vi "SetParam.vi"(8 "error in (no error)":errorcluster caption="entrée d'erreur (pas d'erreur)", 10 "manhattan_distances":cluster{"sum_over_features":bool}={"sum_over_features"=TRUE}, 11 "Manhattan_distances.lvclass":refnum<class "Manhattan_distances.lvclass">) -> (0 "error out":errorcluster caption="sortie d'erreur", 3 "Manhattan_distances.lvclass":refnum<class "Manhattan_distances.lvclass">)   [LabVIEW 2020, in "Manhattan_distances.lvclass"]
doc: "Set Parameters"
uses:
  Manhattan_distances.lvclass
  Manhattan_distances.lvclass/Manhattan_distances.ctl
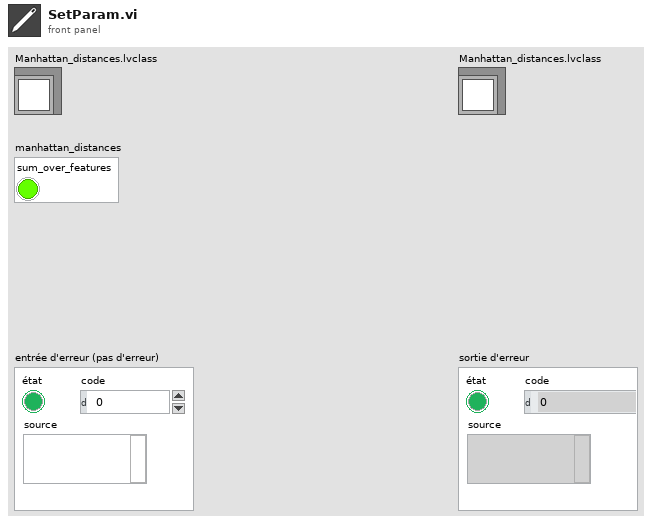
[diagram p1: front panel]
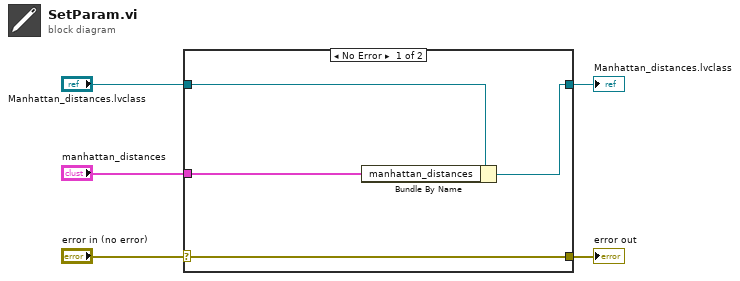
[diagram p0: block diagram]
diagram:
  n1 = case shown="No Error" "error in (no error)" {
    selector: "error in (no error)" -> [w9 w10]
    tunnel: [w9 w10] -> w4
    tunnel: [w7 w11] -> w2
    tunnel: "Manhattan_distances.lvclass" -> [w8 w11]
    tunnel: "manhattan_distances" -> [w6 _]
    frame No Error {
      n2 = Bundle By Name(cluster=w8, "manhattan_distances"=w6) -> (w7:refnum<class "Manhattan_distances.lvclass">)
    }
    frame Error {
    }
  }
  "error out" <- w4
  "Manhattan_distances.lvclass" <- w2
